vi "Write Telemetry Data To DB.vi"(8 "error in (no error)":errorcluster, 10 "Telemetry Data":T1, 11 "Refnum in":T3) -> (0 "error out":errorcluster, 3 "Refnum out":T3)   [LabVIEW 2026, in "Database.lvlib"]
uses:
  Database.lvlib
  <vilib>/addons/database/Connection.llb/Conn ObjectReference.ctl
  Controls/Telemetry_Data_Type.ctl
  Controls/Channels.ctl
  <vilib>/addons/database/Connection.llb/Conn Execute.vi
  <vilib>/addons/database/Recordset.llb/Rec Destroy - Connection.vi
  <vilib>/addons/database/NI_Database_API.lvlib
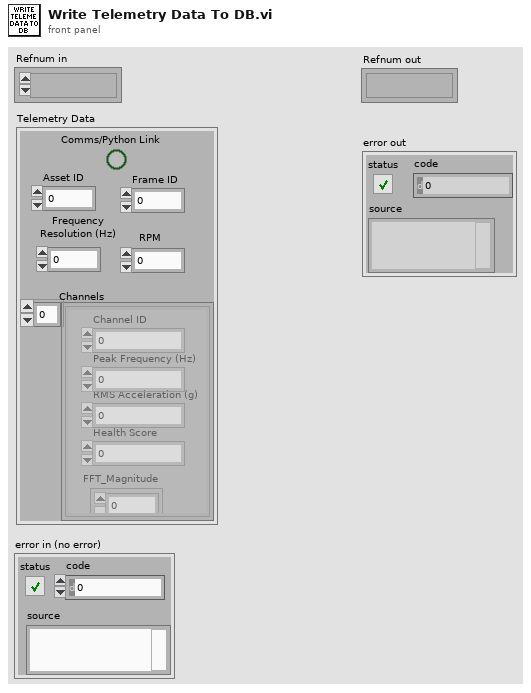
[diagram p1: front panel]
types:
  T1 = typedef "Telemetry_Data_Type.ctl" = cluster{"asset_id":i32, "frame_id":i32, "channels":T2, "comms/python link":bool, "rpm":dbl, "frequency_resolution":dbl}
  T2 = typedef "Channels.ctl" = cluster{"channel_id":dbl, "peak_frequency":dbl, "rms_acceleration":dbl, "health_score":dbl, "fft_magnitude":dbl[]}[]
  T3 = typedef "NI_Database_API.lvlib/Conn ObjectReference.ctl" = refnum<k1>
  T4 = typedef "NI_Database_API.lvlib/Rec ObjectReference.ctl" = refnum<k1>
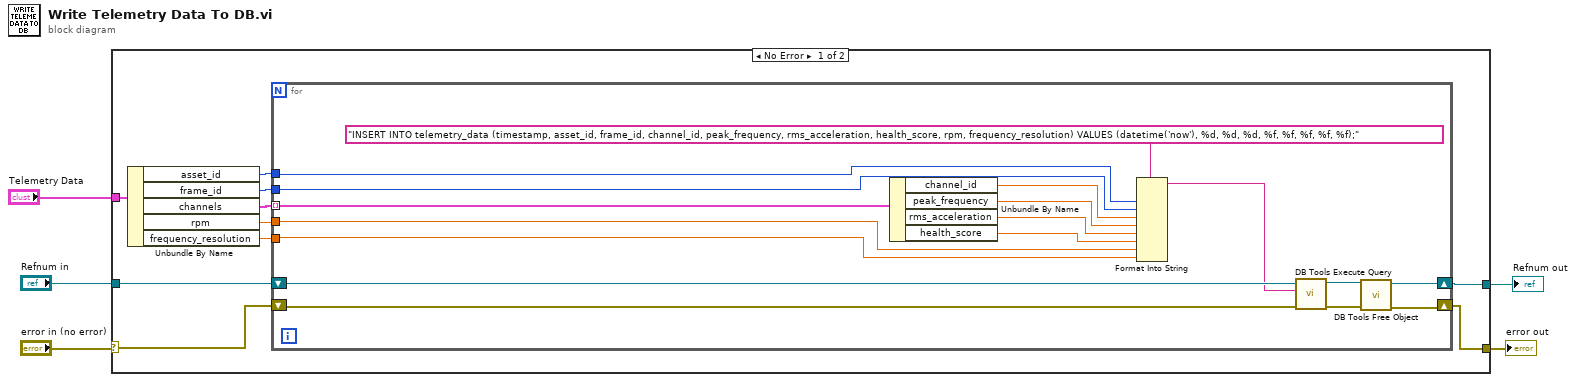
[diagram p0: block diagram]
diagram:
  n1 = case shown="No Error" "error in (no error)" {
    selector: "error in (no error)" -> [w10 w34]
    tunnel: [w8 w34] -> w5
    tunnel: [w9 w33] -> w4
    tunnel: "Refnum in" -> [w11 w33]
    tunnel: "Telemetry Data" -> [w13 _]
    frame No Error {
      n2 = Unbundle By Name(w13) -> ("asset_id"=w12:i32, "frame_id"=w15:i32, "channels"=w14:T2, "rpm"=w7:dbl, "frequency_resolution"=w6:dbl)
      n3 = for {
        tunnel: w14 -> [w32] mode=indexing
        tunnel: w15 -> [w26]
        tunnel: w12 -> [w25]
        shift-right: [w19] -> w8
        shift-left: w10 -> [w22]
        shift-right: [w21] -> w9
        shift-left: w11 -> [w24]
        tunnel: w7 -> [w17]
        tunnel: w6 -> [w16]
        n4 = Unbundle By Name(w32) -> ("channel_id"=w31:dbl, "peak_frequency"=w30:dbl, "rms_acceleration"=w29:dbl, "health_score"=w28:dbl)
        n5 = Format Into String(format string="INSERT INTO telemetry_data (timestamp, asset_id, frame_id, channel_id, peak_frequency, rms_acceleration, health_score, rpm, frequency_resolution) VALUES (datetime('now'), %d, %d, %d, %f, %f, %f, %f, %f);", w25, w26, w31, w30, w29, w28, w17, w16) -> (resulting string=w23:string)  [unwired: 2 in, 1 out]
        n6 = call-poly <vilib>:"DB Tools Execute Query.vi"("error in (no error)"=w22, "SQL query"=w23, "connection reference"=w24) -> ("error out"=w20:errorcluster, "recordset reference"=w18:T4)  [unwired: 5 in]
        n7 = call-poly <vilib>:"DB Tools Free Object.vi"("error in (no error)"=w20, "recordset reference"=w18) -> ("error out"=w19:errorcluster, "connection reference"=w21:T3)  [unwired: 8 in]
      }
    }
    frame Error {
    }
  }
  "error out" <- w5
  "Refnum out" <- w4
